vi "Set VISA User Data.vi"(8 "error in (no error)":errorcluster, 10 "User Data":i32=8, 11 "VISA Refnum in":refnum<visa-resource-name>) -> (0 "error out":errorcluster, 3 "VISA Refnum out":refnum<visa-resource-name>)   [LabVIEW 2019, in "KH7008.lvlib"]
uses:
  KH7008.lvlib
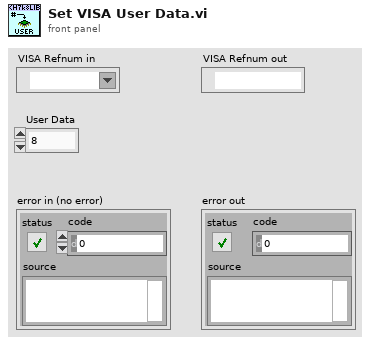
[diagram p1: front panel]
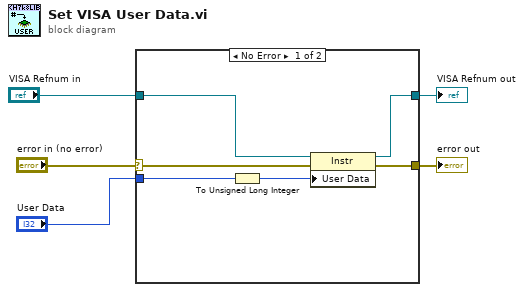
[diagram p0: block diagram]
diagram:
  n1 = case shown="No Error" "error in (no error)" {
    selector: "error in (no error)" -> [w11 w12]
    tunnel: [w10 w12] -> w4
    tunnel: [w9 w13] -> w3
    tunnel: "VISA Refnum in" -> [w8 w13]
    tunnel: "User Data" -> [w7 _]
    frame No Error {
      n2 = To Unsigned Long Integer(number=w7) -> (unsigned 32bit integer=w6:u32)
      n3 = property class="Instr"(reference=w8, error in=w11, "User Data"=w6) -> (reference out=w9:refnum<visa-resource-name>, error out=w10:errorcluster)
    }
    frame Error {
    }
  }
  "error out" <- w4
  "VISA Refnum out" <- w3
